vi "Initialize Network Engine.vi"(8 "error in (no error)":errorcluster, 10 "Parameters":T2 {"Config"."Industrial Settings"."Write Refs"."Data Reference" format="%.0x"; "Config"."Industrial Settings"."Read Refs"."Data Reference" format="%.0x"; "Config"."PID Settings"."Read Refs"."Data Reference" format="%.0x"; "Config"."PID Settings"."Write Refs"."Data Reference" format="%.0x"}, 11 "Process":refnum<class "Process.lvclass">) -> (0 "error out":errorcluster, 2 "Start":bool, 3 "State Variables":T1)   [LabVIEW 2019, in "Control Addon Engine.lvlib"]
uses:
  Control Addon Engine.lvlib
  Types/RT Configuration.ctl
  Addon Shared/Types/Gain Schedule.ctl
  Addon Shared/Types/Compiled Settings.ctl
  Addon Shared/Types/Compiled PID Settings.ctl
  <vilib>/NI VeriStand/Custom Device API/Block Data Reference.ctl
  <vilib>/NI VeriStand/Custom Device API/Data Reference.ctl
  Addon Shared/Types/Compiled Industrial Settings.ctl
  Addon Shared/Types/Compiled Industrial Parameters.ctl
  Types/Network Engine State Variables.ctl
  <vilib>/NI/NIVS Inline Async API/_VS Inline Async API/Process/Process.lvclass
  <vilib>/NI/NI VeriStand Addon Network Comm/Engine/VeriStand Comm.lvclass
  <vilib>/NI/NI VeriStand Addon Network Comm/Engine/VeriStand Comm.lvclass/VeriStand Comm.ctl
  <vilib>/NI/NIVS Inline Async API/_VS Inline Async API/Process/Process.lvclass/Process.ctl
  <vilib>/NI/NIVS Inline Async API/_VS Inline Async API/Error Handling Process/SubVIs/Error.ConvertArray.vi
  <vilib>/Utility/SystemLogging/Write to System Log.vi
  <vilib>/NI/AMC/Create Message Queue.vi
  <vilib>/NI/STM/Connection Manager/TCP/Advanced/TCP Initialize Connection Manager (By Reference).vi
  Addon Shared/Control Addon Shared.lvlib
  <vilib>/NI VeriStand/Custom Device API/Custom Device API.lvlib
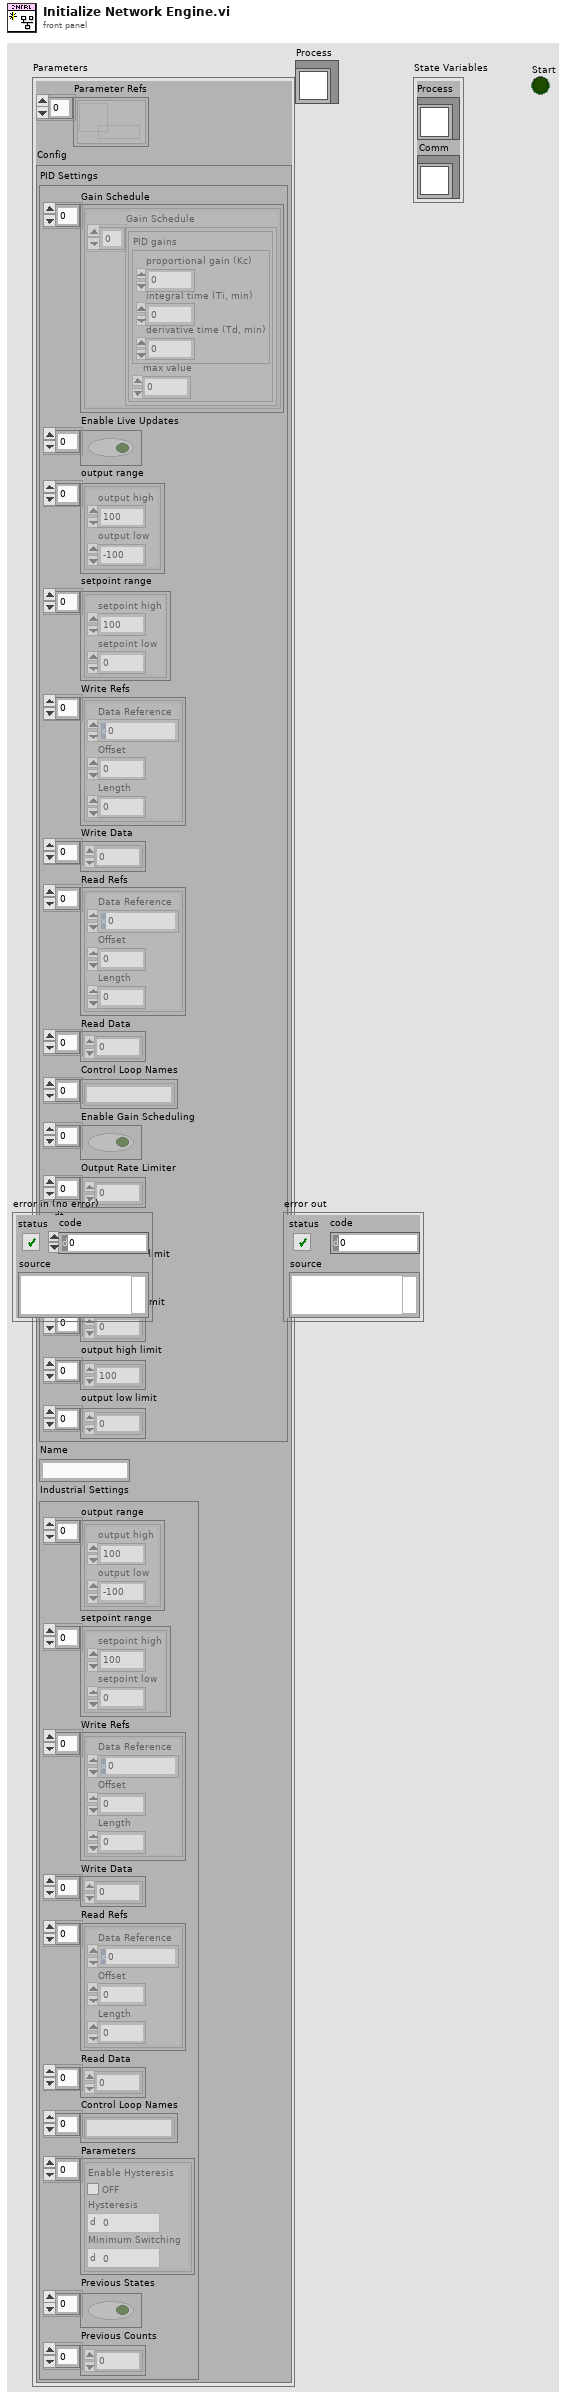
[diagram p1: front panel]
types:
  T1 = typedef "Control Addon Engine.lvlib/Network Engine State Variables.ctl" = cluster{"Process":refnum<class "Process.lvclass">, "Comm":refnum<class "VeriStand Comm.lvclass">}
  T2 = typedef "Control Addon Engine.lvlib/RT Configuration.ctl" = cluster{"Parameter Refs":refnum<data-value>[], "Config":T3}
  T3 = typedef "Control Addon Shared.lvlib/Compiled Settings.ctl" = cluster{"PID Settings":T4, "Name":string, "Industrial Settings":T8}
  T4 = typedef "Control Addon Shared.lvlib/Compiled PID Settings.ctl" = cluster{"Gain Schedule":T5[], "Enable Live Updates":bool[], "output range":cluster{"output high":dbl, "output low":dbl}[], "setpoint range":cluster{"setpoint high":dbl, "setpoint low":dbl}[], "Write Refs":T6[], "Write Data":dbl[], "Read Refs":T6[], "Read Data":dbl[], "Control Loop Names":string[], "Enable Gain Scheduling":bool[], "Output Rate Limiter":dbl[], "dt":dbl, "setpoint high limit":dbl[], "setpoint low limit":dbl[], "output high limit":dbl[], "output low limit":dbl[]}
  T5 = typedef "Control Addon Shared.lvlib/Gain Schedule.ctl" = cluster{"Gain Schedule":cluster{"PID gains":cluster{"proportional gain (Kc)":dbl, "integral time (Ti, min)":dbl, "derivative time (Td, min)":dbl}, "max value":dbl}[]}
  T6 = typedef "Custom Device API.lvlib/Block Data Reference.ctl" = cluster{"Data Reference":T7, "Offset":u64, "Length":u64}
  T7 = typedef "Custom Device API.lvlib/Data Reference.ctl" = i32
  T8 = typedef "Control Addon Shared.lvlib/Compiled Industrial Settings.ctl" = cluster{"output range":cluster{"output high":dbl, "output low":dbl}[], "setpoint range":cluster{"setpoint high":dbl, "setpoint low":dbl}[], "Write Refs":T6[], "Write Data":dbl[], "Read Refs":T6[], "Read Data":dbl[], "Control Loop Names":string[], "Parameters":T9[], "Previous States":bool[], "Previous Counts":u64[]}
  T9 = typedef "Control Addon Shared.lvlib/Compiled Industrial Parameters.ctl" = cluster{"Enable Hysteresis":bool, "Hysteresis":dbl, "Minimum Switching":u64}
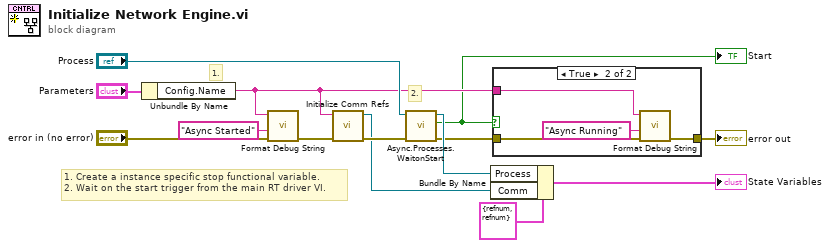
[diagram p0: block diagram]
diagram:
  # "1. Create a instance specific stop functional variable.\n2. Wait on the start trigger from the main RT driver VI."
  # "2."
  # "1."
  n1 = Unbundle By Name("Parameters") -> ("Config.Name"=w2:string)
  n2 = call "Format Debug String.vi"("error in (no error)"="error in (no error)", "State"="Async Started", "Name"=w2) -> ("error out"=w6:errorcluster)  [unwired: 8 in]
  n3 = call <vilib>:"Initialize Comm Refs.vi"("error in (no error)"=w6, "Name"=w2) -> ("error out"=w12:errorcluster, "Comm.lvclass"=w8:refnum<class "VeriStand Comm.lvclass">)  [unwired: 8 in]
  n4 = call <vilib>:"Async.Processes.WaitonStart.vi"("error in (no error)"=w12, "Process"="Process") -> ("error out"=w4:errorcluster, "Execute"=w1:bool, "Process out"=w10:refnum<class "Process.lvclass">)  [unwired: 7 in]
  "Start" <- w1
  n5 = Bundle By Name(cluster=T1 {"Process"=refnum, "Comm"=refnum} ("State Variables"), "Process"=w10, "Comm"=w8) -> (→"State Variables":T1)
  n6 = case shown="True" w1 {
    tunnel: w4 -> [w15 w18]
    tunnel: [w15 w17] -> w3
    tunnel: w2 -> [_ w16]
    frame False {
    }
    frame True {
      n7 = call "Format Debug String.vi"("error in (no error)"=w18, "State"="Async Running", "Name"=w16) -> ("error out"=w17:errorcluster)  [unwired: 8 in]
    }
  }
  "error out" <- w3
